vi "题目1.vi"   [LabVIEW 2017]
types:
  T1 = enum16{"open", "replace", "create", "open or create", "replace or create", "replace or create with confirmation"}
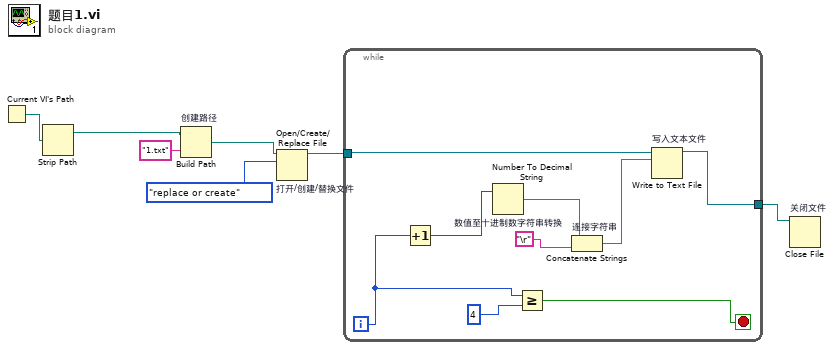
[diagram p0: block diagram]
diagram:
  n1 = Current VI's Path() -> (path=w2:path)
  n2 = Strip Path(path=w2) -> (stripped path=w3:path)  [unwired: 1 out]
  n3 = Build Path "创建路径"(base path=w3, name or relative path="1.txt" ("名称或相对路径")) -> (appended path=w5:path)
  n4 = Open/Create/Replace File "打开/创建/替换文件"(file path (use dialog)=w5, operation (0:open)=T1."replace or create" ("操作(0:open)")) -> (refnum out=w7:refnum<file>)  [unwired: 4 in, 2 out]
  n5 = while {
    tunnel: w7 -> [w10]
    tunnel: [w8] -> w1
    i -> [w12]
    stop <- w9 stop-if-true
    n6 = Increment(x=w12) -> (x+1=w16:i32)
    n7 = Number To Decimal String "数值至十进制数字符串转换"(number=w16) -> (decimal integer string=w15:string)  [unwired: 1 in]
    n8 = Greater Or Equal?(x=w12, y=4) -> (x >= y?=w9:bool)
    n9 = Concatenate Strings "连接字符串"(w15, "\r") -> (w13:string)
    n10 = Write to Text File "写入文本文件"(file (use dialog)=w10, text=w13) -> (refnum out=w8:refnum<file>)  [unwired: 2 in, 2 out]
  }
  n11 = Close File "关闭文件"(refnum=w1) -> ()  [unwired: 1 in, 2 out]
